vi "Write Command FIFO.vi"(8 "error in (no error)":errorcluster, 9 "timeout in ms (0)":i32 format="%d ms", 10 "command":T1, 11 "Thread in":refnum<class "Thread.lvclass">) -> (0 "error out":errorcluster, 1 "timed out?":bool, 3 "Thread out":refnum<class "Thread.lvclass">, 4 "# elements":u32)   [LabVIEW 2019, in "DSF Core.lvlib" / "Thread.lvclass"]
uses:
  Thread.lvclass
  Thread Command.ctl
  Thread.lvclass/Thread.ctl
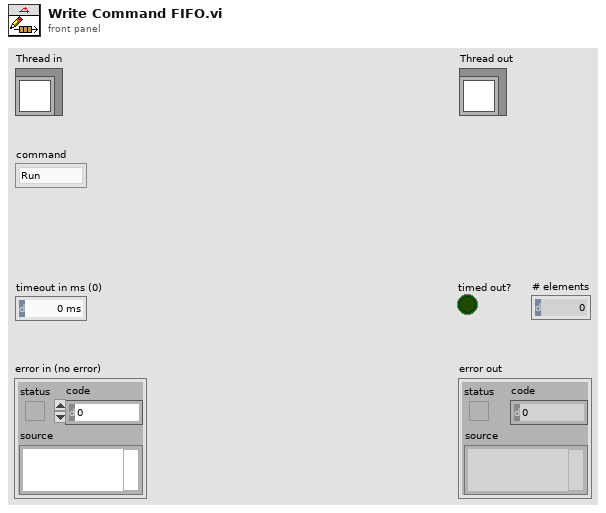
[diagram p1: front panel]
types:
  T1 = typedef "DSF Core.lvlib/Thread.lvclass/Thread Command.ctl" = enum8{"Run", "Shutdown"}
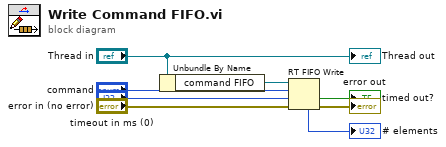
[diagram p0: block diagram]
diagram:
  n1 = Unbundle By Name("Thread in") -> ("command FIFO"=w5:refnum<k33>)
  n2 = RT FIFO Write(0:w5, 1:"command", 2:"timeout in ms (0)", 3:"error in (no error)") -> (7:→"# elements":u32, 10:→"timed out?":bool, 11:→"error out":errorcluster)  [unwired: 1 in, 1 out]
  "Thread out" <- "Thread in"
